vi "Singleton Test.vi"() -> ()   [LabVIEW 2017]
uses:
  Single Object/SingleObject.lvclass/SingleObject.ctl
  Single Object/SingleObject.lvclass
panel:
  in  "stop":bool
  in  "Show Message":bool
  in  "Message":string
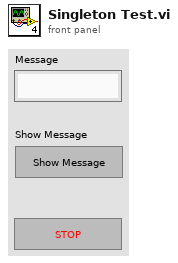
[diagram p1: front panel]
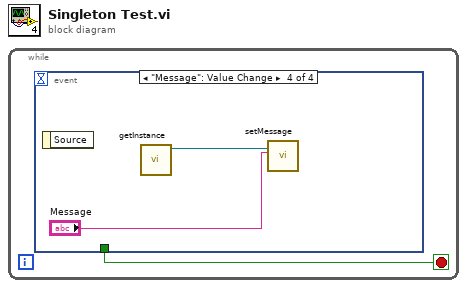
[diagram p0: block diagram]
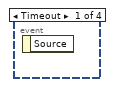
[diagram p2: hidden frame]
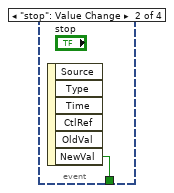
[diagram p3: hidden frame]
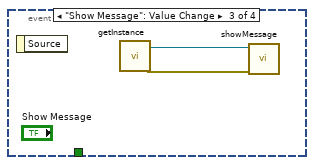
[diagram p4: hidden frame]
diagram:
  n1 = while {
    stop <- w1 stop-if-true
    n2 = event shown="[3] \"Message\": Value Change" {
      selector: _ -> [_ _ _ _]
      dyn-events: _ -> [_ _ _ _]
      timeout: _ -> [_ _ _ _]
      tunnel: [_ w2 _ _] -> w1
      event Timeout {
        n3 = event-data() -> ()  [unwired: 1 in, 1 out]
      }
      event "stop": Value Change {
        n4 = event-data() -> ("NewVal"=w2:bool)  [unwired: 1 in, 5 out]
      }
      event "Show Message": Value Change {
        n5 = event-data() -> ()  [unwired: 1 in, 1 out]
        n6 = call "getInstance.vi"() -> ("error out"=w3:errorcluster, "Instance out"=w4:refnum<data-value>)  [unwired: 10 in]
        n7 = call "showMessage.vi"("error in (no error)"=w3, "Instance In"=w4) -> ()  [unwired: 8 in, 2 out]
      }
      event "Message": Value Change {
        n8 = event-data() -> ()  [unwired: 1 in, 1 out]
        n9 = call "getInstance.vi"() -> ("Instance out"=w6:refnum<data-value>)  [unwired: 10 in, 1 out]
        n10 = call "setMessage.vi"("Message"="Message", "Instance In"=w6) -> ()  [unwired: 8 in, 2 out]
      }
    }
  }
